vi "ActiView806-Lores.vi"() -> ()   [LabVIEW 2020] (continued)
                        i -> [w570]
                        n163 = call-poly <vilib>:"Read Key.vi"("section"=w578, "error in (no error)"=w588, "key"=w573, "refnum"=w589) -> ("error out"=w576:errorcluster, "value"=w584:string, "found?"=w583:bool, "refnum out"=w577:T19)  [unwired: 2 in, 2 out]
                        n164 = Decimal String To Number(string=w584) -> (number=w590:i32)  [unwired: 3 out]
                        n165 = Not(x=w583) -> (.not. x?=w586:bool)
                        n166 = Equal?(x="", y=w584) -> (x = y?=w585:bool)
                        n167 = To Byte Integer(number=w590) -> (8bit integer=w569:i8)
                        n168 = Equal To 0?(x=w570) -> (x = 0?=w580:bool)
                        n169 = Or(x=w586, y=w585) -> (x .or. y?=w582:bool)
                        n170 = Not Equal To 0?(x=w569) -> (x != 0?=w581:bool)
                        n171 = And(x=w581, y=w580) -> (x .and. y?=w579:bool)
                        n172 = case shown="True" w579 {
                          tunnel: w573 -> [_ w609]
                          tunnel: w578 -> [_ w608]
                          tunnel: w577 -> [w600 w607]
                          tunnel: w576 -> [w601 w606]
                          tunnel: w574 -> [_ w605]
                          tunnel: [w601 w604] -> w572
                          tunnel: [w600 w603] -> w575
                          frame False {
                          }
                          frame True {
                            n173 = call "Act_Warning.vi"() -> ("Warning?"=w602:bool)  [unwired: 1 out]
                            n174 = case shown="False" w602 {
                              tunnel: w609 -> [w615 _]
                              tunnel: w608 -> [w617 _]
                              tunnel: w607 -> [w616 w633]
                              tunnel: w606 -> [w610 w634]
                              tunnel: w605 -> [w614 _]
                              tunnel: [w612 w634] -> w604
                              tunnel: [w611 w633] -> w603
                              frame False {
                                n175 = flat-sequence {
                                tunnel: w617 -> [w628]
                                tunnel: w610 -> [w627]
                                tunnel: w616 -> [w626]
                                tunnel: w615 -> [w625]
                                tunnel: [w619] -> w613
                                tunnel: w614 -> [w632]
                                tunnel: w613 -> [w631]
                                tunnel: [w629] -> w612
                                tunnel: [w630] -> w611
                                frame #0 {
                                w618 = "0"  # No Warning
                                w620 = T18 1 items=["no dialog", "OK message", "continue or stop message", "OK message + warnings", "continue/stop + warnings"] ("type of dialog (OK msg:1)")
                                w623 = TRUE  # write configuration file? (T)
                                n176 = call-poly <vilib>:"Write Key.vi"("section"=w628, "error in (no error)"=w627, "value"=w618, "key"=w625, "refnum"=w626) -> ("error out"=w621:errorcluster, "refnum out"=w622:T19)  [unwired: 1 in, 4 out]
                                n177 = call <vilib>:"Close Config Data.vi"("error in (no error)"=w621, "write file if changed (T)"=w623, "refnum"=w622) -> ("error out"=w624:errorcluster)  [unwired: 8 out]
                                n178 = call <vilib>:"General Error Handler.vi"("type of dialog (OK msg:1)"=w620, "error in (no error)"=w624) -> ("error out"=w619:errorcluster)  [unwired: 1 in, 12 out]
                                }
                                frame #1 {
                                n179 = call <vilib>:"Open Config Data.vi"("error in (no error)"=w631, "configuration file path"=w632) -> ("error out"=w629:errorcluster, "refnum"=w630:T19)  [unwired: 7 in, 1 out]
                                }
                                }
                              }
                              frame True {
                              }
                            }
                          }
                        }
                        n180 = case shown="0, Default" w570 {
                          tunnel: w569 -> [w591 w595 w599]
                          tunnel: [w591 w592 w596] -> w571
                          frame 0, Default {
                          }
                          frame 4 {
                            # "LineWidth"
                            n181 = In Range and Coerce(upper limit=i8 1, x=w595, lower limit=i8 5) -> (coerced(x)=w592:i8)  [unwired: 1 out]
                          }
                          frame 5 {
                            # "Cursor"
                            n182 = In Range and Coerce(upper limit=i8 0, x=w599, lower limit=i8 1) -> (coerced(x)=w596:i8)  [unwired: 1 out]
                          }
                        }
                      }
                      n183 = Index Array(array=w557, index #1=2 ("index"), index #2=4 ("index")) -> (element #1=w554:i8, element #2=w558:i8)
                      n184 = To Unsigned Byte Integer(number=w558) -> (unsigned 8bit integer=w556:u8)
                      n185 = Or Array Elements(Boolean array=w561) -> (logical OR=w568:bool)
                    }
                    frame #1 {
                      # "Not Found"
                      # "Vbat is not a trace"
                      n186 = Decrement(x=w657) -> (x-1=w635:i32)
                      n187 = Add(x=w652, y=w642) -> (x+y=w641:i32)
                      n188 = Add(x=w652, y=w642) -> (x+y=w653:i32)
                      n189 = Add(x=w641, y=w657) -> (x+y=w640:i32)
                      n190 = Add(x=w640, y=w636) -> (x+y=w639:i32)
                      n191 = Add(x=w639, y=w650) -> (x+y=w655:i32)
                      n192 = for {
                        N: w653 -> [_]
                        tunnel: w649 -> [w751]
                        i -> [w750]
                        n193 = To Unsigned Long Integer(number=w750) -> (unsigned 32bit integer=w749:u32)
                        n194 = property on="Mon Chart" class="WFChart (strict)"("Active Plot"=w749, "Plot.Line Width"=w751) -> ()  [unwired: 2 in, 2 out]
                      }
                      n195 = for {
                        N: w652 -> [_]
                        tunnel: w649 -> [w748]
                        i -> [w747]
                        n196 = To Unsigned Long Integer(number=w747) -> (unsigned 32bit integer=w746:u32)
                        n197 = property on="Bip Chart" class="WFChart (strict)"("Active Plot"=w746, "Plot.Line Width"=w748) -> ()  [unwired: 2 in, 2 out]
                      }
                      n198 = To Unsigned Long Integer(number=w653) -> (unsigned 32bit integer=w671:u32)
                      n199 = To Unsigned Long Integer(number=w652) -> (unsigned 32bit integer=w660:u32)
                      n200 = To Unsigned Long Integer(number=w635) -> (unsigned 32bit integer=w659:u32)
                      n201 = To Unsigned Long Integer(number=w636) -> (unsigned 32bit integer=w651:u32)
                      n202 = To Unsigned Long Integer(number=w650) -> (unsigned 32bit integer=w656:u32)
                      n203 = Increment(x=w655) -> (x+1=w645:i32)
                      n204 = for {
                        N: w645 -> [w684]
                        shift-right: [w705] -> w644
                        shift-left: w647 -> [w707]
                        shift-right: [w704] -> w643
                        shift-left: w646 -> [w706]
                        tunnel: [w681] -> w637 mode=indexing
                        tunnel: [w693] -> w638 mode=indexing
                        tunnel: w642 -> [w685]
                        tunnel: w641 -> [w696]
                        tunnel: w648 -> [w680]
                        tunnel: w640 -> [w686]
                        tunnel: w639 -> [w673]
                        i -> [w675]
                        n205 = Increment(x=w675) -> (x+1=w683:i32)
                        n206 = Greater Or Equal?(x=w675, y=w696) -> (x >= y?=w701:bool)
                        n207 = Greater Or Equal?(x=w675, y=w685) -> (x >= y?=w703:bool)
                        n208 = Greater Or Equal?(x=w675, y=w686) -> (x >= y?=w687:bool)
                        n209 = Greater Or Equal?(x=w675, y=w673) -> (x >= y?=w674:bool)
                        n210 = Select(t=i8 1, s=w703, f=i8 0) -> (s? t:f=w702:i8)
                        n211 = Equal?(x=w684, y=w683) -> (x = y?=w676:bool)
                        n212 = Select(t=i8 2, s=w701, f=w702) -> (s? t:f=w690:i8)
                        n213 = Select(t=i8 3, s=w687, f=w690) -> (s? t:f=w689:i8)
                        n214 = Select(t=i8 4, s=w674, f=w689) -> (s? t:f=w678:i8)
                        n215 = Select(t=i8 5, s=w676, f=w678) -> (s? t:f=w679:i8)
                        n216 = case shown="5" w679 {
                          tunnel: [w711 w717 w723 w729 w735 "Trig" ("string")] -> w682
                          tunnel: w683 -> [w708 w715 w722 w726 w732 _]
                          tunnel: w685 -> [_ w714 _ _ _ _]
                          tunnel: w696 -> [_ _ w720 _ _ _]
                          tunnel: w686 -> [_ _ _ w724 _ _]
                          tunnel: w673 -> [_ _ _ _ w730 _]
                          frame 0, Default {
                            n217 = Number To Decimal String(number=w708) -> (decimal integer string=w709:string)  [unwired: 1 out]
                            n218 = Concatenate Strings("Chan" ("string"), w709) -> (w711:string)
                          }
                          frame 1 {
                            n219 = Subtract(x=w715, y=w714) -> (x-y=w712:i32)
                            n220 = Number To Decimal String(number=w712) -> (decimal integer string=w713:string)  [unwired: 1 out]
                            n221 = Concatenate Strings("Tou" ("string"), w713) -> (w717:string)
                          }
                          frame 2 {
                            n222 = Subtract(x=w722, y=w720) -> (x-y=w718:i32)
                            n223 = Number To Decimal String(number=w718) -> (decimal integer string=w719:string)  [unwired: 1 out]
                            n224 = Concatenate Strings("Aux" ("string"), w719) -> (w723:string)
                          }
                          frame 3 {
                            n225 = Subtract(x=w726, y=w724) -> (x-y=w725:i32)
                            n226 = Number To Decimal String(number=w725) -> (decimal integer string=w727:string)  [unwired: 1 out]
                            n227 = Concatenate Strings("Jazz" ("string"), w727) -> (w729:string)
                          }
                          frame 4 {
                            n228 = Subtract(x=w732, y=w730) -> (x-y=w731:i32)
                            n229 = Number To Decimal String(number=w731) -> (decimal integer string=w733:string)  [unwired: 1 out]
                            n230 = Concatenate Strings("Box" ("string"), w733) -> (w735:string)
                          }
                          frame 5 {
                          }
                        }
                        n231 = call-poly <vilib>:"Read Key.vi"("section"=w680, "error in (no error)"=w706, "key"=w682, "refnum"=w707) -> ("error out"=w704:errorcluster, "value"=w681:string, "found?"=w695:bool, "refnum out"=w705:T19)  [unwired: 2 in, 2 out]
                        n232 = Equal?(x="", y=w681) -> (x = y?=w691:bool)
                        n233 = Not(x=w695) -> (.not. x?=w694:bool)
                        n234 = Or(x=w691, y=w694) -> (x .or. y?=w693:bool)
                      }
                      n235 = property on="Mon Chart" class="WFChart (strict)"("Legend:Plots Shown"=w671) -> ()  [unwired: 2 in, 2 out]
                      n236 = property on="Bip Chart" class="WFChart (strict)"("Legend:Plots Shown"=w660) -> ()  [unwired: 2 in, 2 out]
                      n237 = property on="Aux Chart" class="WFChart (strict)"("Legend:Plots Shown"=w659) -> ()  [unwired: 2 in, 2 out]
                      n238 = property on="Jazz Chart" class="WFChart (strict)"("LegPlots"=w651) -> ()  [unwired: 2 in, 2 out]
                      n239 = property on="Ana Chart" class="WFChart (strict)"("Legend:Plots Shown"=w656) -> ()  [unwired: 2 in, 2 out]
                      n240 = Or Array Elements(Boolean array=w638) -> (logical OR=w654:bool)
                      n241 = Quotient & Remainder(x=w642, y=2) -> (floor(x/y)=w661:i32)  [unwired: 1 out]
                      n242 = case shown="False" w654 {
                        tunnel: w641 -> [w763 _]
                        tunnel: w652 -> [w762 _]
                        tunnel: w635 -> [w761 _]
                        tunnel: w642 -> [w760 _]
                        tunnel: w639 -> [w759 _]
                        tunnel: w650 -> [w758 _]
                        tunnel: w637 -> [w754 _]
                        tunnel: w636 -> [w756 _]
                        tunnel: w640 -> [w753 _]
                        frame False {
                          n243 = for {
                            N: w761 -> [_]
                            tunnel: w754 -> [w780]
                            tunnel: w763 -> [w781]
                            tunnel: [w779] -> w752 mode=indexing
                            i -> [w783]
                            n244 = Add(x=w781, y=w783) -> (x+y=w784:i32)
                            n245 = Index Array(array=w780, index=w784) -> (element=w785:string)
                            n246 = String Subset(string=w785, length (rest)=4 ("length (rest)")) -> (substring=w779:string)  [unwired: 1 out]
                          }
                          n247 = for {
                            N: w756 -> [_]
                            tunnel: w754 -> [w766]
                            tunnel: w753 -> [w767]
                            tunnel: [w765] -> w755 mode=indexing
                            i -> [w769]
                            n248 = Add(x=w767, y=w769) -> (x+y=w770:i32)
                            n249 = Index Array(array=w766, index=w770) -> (element=w771:string)
                            n250 = String Subset(string=w771, length (rest)=4 ("length (rest)")) -> (substring=w765:string)  [unwired: 1 out]
                          }
                          n251 = for {
                            N: w758 -> [_]
                            tunnel: w754 -> [w773]
                            tunnel: w759 -> [w774]
                            tunnel: [w772] -> w757 mode=indexing
                            i -> [w776]
                            n252 = Add(x=w774, y=w776) -> (x+y=w777:i32)
                            n253 = Index Array(array=w773, index=w777) -> (element=w778:string)
                            n254 = String Subset(string=w778, length (rest)=8 ("length (rest)")) -> (substring=w772:string)  [unwired: 1 out]
                          }
                          n255 = for {
                            N: w762 -> [w793]
                            tunnel: w754 -> [w798]
                            tunnel: w760 -> [w791]
                            tunnel: [w794] -> w764 mode=indexing
                            i -> [w789]
                            w786 = 4 ("length (rest)")
                            n256 = Increment(x=w789) -> (x+1=w788:i32)
                            n257 = Quotient & Remainder(x=w788, y=w793) -> (x-y*floor(x/y)=w787:i32)  [unwired: 1 out]
                            n258 = Add(x=w791, y=w789) -> (x+y=w792:i32)
                            n259 = Add(x=w791, y=w787) -> (x+y=w790:i32)
                            n260 = Index Array(array=w798, index=w792) -> (element=w800:string)
                            n261 = Index Array(array=w798, index=w790) -> (element=w799:string)
                            n262 = String Subset(string=w799, length (rest)=w786) -> (substring=w796:string)  [unwired: 1 out]
                            n263 = String Subset(string=w800, length (rest)=w786) -> (substring=w797:string)  [unwired: 1 out]
                            n264 = Concatenate Strings(w797, "-" ("string"), w796) -> (w794:string)
                          }
                          n265 = property on="AuxFree" class="LstBox (strict)"("Item Names"=w752) -> ()  [unwired: 2 in, 2 out]
                          n266 = property on="JazzFree" class="LstBox (strict)"("Item Names"=w755) -> ()  [unwired: 2 in, 2 out]
                          n267 = property on="AnaFree" class="LstBox (strict)"("Item Names"=w757) -> ()  [unwired: 2 in, 2 out]
                          n268 = property on="AnaOffset" class="Ring (strict)"("Strings []"=w757) -> ()  [unwired: 2 in, 2 out]
                          n269 = property on="BipFree" class="LstBox (strict)"("Item Names"=w764) -> ()  [unwired: 2 in, 2 out]
                        }
                        frame True {
                        }
                      }
                      n270 = Increment(x=w661) -> (x+1=w669:i32)
                      n271 = Increment(x=w661) -> (x+1=w664:i32)
                      n272 = for {
                        N: w636 -> [_]
                        tunnel: w649 -> [w739]
                        i -> [w738]
                        n273 = To Unsigned Long Integer(number=w738) -> (unsigned 32bit integer=w737:u32)
                        n274 = property on="Jazz Chart" class="WFChart (strict)"("Active Plot"=w737, "Plot.Line Width"=w739) -> ()  [unwired: 2 in, 2 out]
                      }
                      n275 = for {
                        N: w635 -> [_]
                        tunnel: w649 -> [w745]
                        i -> [w744]
                        n276 = To Unsigned Long Integer(number=w744) -> (unsigned 32bit integer=w743:u32)
                        n277 = property on="Aux Chart" class="WFChart (strict)"("Active Plot"=w743, "Plot.Line Width"=w745) -> ()  [unwired: 2 in, 2 out]
                      }
                      n278 = Increment(x=w664) -> (x+1=w670:i32)
                      n279 = Increment(x=w669) -> (x+1=w666:i32)
                      n280 = for {
                        N: w670 -> [w807]
                        tunnel: [w803] -> w663 mode=indexing
                        tunnel: [w801] -> w665
                        i -> [w810]
                        w801 = 1.0 ("X Scale.Offset and Multiplier:Offset")
                        w811 = 0.5 ("f")
                        n281 = Decrement(x=w807) -> (x-1=w806:i32)
                        n282 = Equal To 0?(x=w810) -> (x = 0?=w813:bool)
                        n283 = Equal?(x=w806, y=w810) -> (x = y?=w809:bool)
                        n284 = To Double Precision Float(number=w810) -> (double precision float=w812:dbl)
                        n285 = To Double Precision Float(number=w806) -> (double precision float=w805:dbl)
                        n286 = Select(t=w811, s=w813, f=w812) -> (s? t:f=w808:dbl)
                        n287 = Subtract(x=w805, y=w811) -> (x-y=w804:dbl)
                        n288 = Select(t=w804, s=w809, f=w808) -> (s? t:f=w802:dbl)
                        n289 = Subtract(x=w802, y=w801) -> (x-y=w803:dbl)
                      }
                      n290 = for {
                        N: w666 -> [w821]
                        tunnel: [w814] -> w667 mode=indexing
                        tunnel: [w816] -> w668
                        tunnel: w669 -> [w817]
                        i -> [w824]
                        w825 = 0.5 ("f")
                        n291 = Decrement(x=w821) -> (x-1=w820:i32)
                        n292 = Equal To 0?(x=w824) -> (x = 0?=w827:bool)
                        n293 = Equal?(x=w820, y=w824) -> (x = y?=w823:bool)
                        n294 = To Double Precision Float(number=w824) -> (double precision float=w826:dbl)
                        n295 = To Double Precision Float(number=w820) -> (double precision float=w819:dbl)
                        n296 = Select(t=w825, s=w827, f=w826) -> (s? t:f=w822:dbl)
                        n297 = Subtract(x=w819, y=w825) -> (x-y=w818:dbl)
                        n298 = To Double Precision Float(number=w817) -> (double precision float=w816:dbl)
                        n299 = Select(t=w818, s=w823, f=w822) -> (s? t:f=w815:dbl)
                        n300 = Decrement(x=w815) -> (x-1=w814:dbl)
                      }
                      n301 = for {
                        N: w650 -> [_]
                        tunnel: w649 -> [w742]
                        i -> [w741]
                        n302 = To Unsigned Long Integer(number=w741) -> (unsigned 32bit integer=w740:u32)
                        n303 = property on="Ana Chart" class="WFChart (strict)"("Active Plot"=w740, "Plot.Line Width"=w742) -> ()  [unwired: 2 in, 2 out]
                      }
                      n304 = property on="Offset Graph First Half" class="WFGraph (strict)"("X Scale.Marker Values[]"=w663) -> ()  [unwired: 2 in, 2 out]
                      n305 = property on="Offset Graph  Second Half" class="WFGraph (strict)"("X Scale.Marker Values[]"=w667) -> ()  [unwired: 2 in, 2 out]
                      n306 = Bundle By Name(cluster=w672, "All Labels"=w637) -> (w658:T8)
                      n307 = property on="Offset Graph First Half" class="WFGraph (strict)"("X Scale.Offset and Multiplier:Offset"=w665) -> ()  [unwired: 2 in, 2 out]
                      n308 = property on="Offset Graph  Second Half" class="WFGraph (strict)"("X Scale.Offset and Multiplier:Offset"=w668) -> ()  [unwired: 2 in, 2 out]
                    }
                    frame #2 {
                      # "not found"
                      n309 = for {
                        shift-right: [w961] -> w835
                        shift-left: w837 -> [w959]
                        shift-right: [w960] -> w834
                        shift-left: w836 -> [w958]
                        tunnel: [w957] -> w833 mode=indexing
                        tunnel: w830 -> [w956] mode=indexing
                        tunnel: [w950] -> w832 mode=indexing
                        tunnel: w829 -> [w949]
                        n310 = call-poly <vilib>:"Read Key.vi"("section"=w949, "error in (no error)"=w958, "key"=w956, "refnum"=w959) -> ("error out"=w960:errorcluster, "value"=w954:string, "found?"=w955:bool, "refnum out"=w961:T19)  [unwired: 2 in, 2 out]
                        n311 = Decimal String To Number(string=w954) -> (number=w957:i32)  [unwired: 3 out]
                        n312 = Not(x=w955) -> (.not. x?=w952:bool)
                        n313 = Equal?(x="", y=w954) -> (x = y?=w951:bool)
                        n314 = Or(x=w952, y=w951) -> (x .or. y?=w950:bool)
                      }
                      n315 = Or Array Elements(Boolean array=w832) -> (logical OR=w831:bool)
                      n316 = case shown="False" w831 {
                        tunnel: w833 -> [w946 _]
                        tunnel: w828 -> [w853 _]
                        frame False {
                          n317 = Index Array(array=w946) -> (element #1=w838:i32, element #2=w839:i32, element #3=w840:i32, element #4=w841:i32, element #5=w842:i32, element #6=w843:i32, element #7=w844:i32, element #8=w845:i32, element #9=w846:i32, element #10=w847:i32, element #11=w848:i32, element #12=w849:i32, element #13=w850:i32, element #14=w866:i32, element #15=w865:i32, element #16=w860:i32, element #17=w861:i32, element #18=w862:i32, element #19=w863:i32, element #20=w864:i32, element #21=w916:i32, element #22=w915:i32, element #23=w910:i32, element #24=w907:i32, element #25=w906:i32, element #26=w903:i32, element #27=w901:i32, element #28=w888:i32, element #29=w899:i32, element #30=w895:i32, element #31=w894:i32, element #32=w893:i32, element #33=w892:i32, element #34=w891:i32, element #35=w885:i32, element #36=w884:i32, element #37=w883:i32, element #38=w882:i32, element #39=w881:i32, element #40=w871:i32, element #41=w870:i32, element #42=w872:i32, element #43=w873:i32, element #44=w874:i32, element #45=w875:i32, element #46=w876:i32, element #47=w877:i32, element #48=w878:i32)  [unwired: 48 in]
                          n318 = case shown="0, Default" w853 {
                            tunnel: [i32[] [4] ("Disabled Items []") i32[] [] ("Disabled Items []")] -> w852
                            frame 0, Default {
                            }
                            frame 1 {
                            }
                          }
                          n319 = To Double Precision Float(number=w876) -> (double precision float=w926:dbl)
                          n320 = Not Equal To 0?(x=w881) -> (x != 0?=w930:bool)
                          n321 = Not Equal To 0?(x=w899) -> (x != 0?=w900:bool)
                          n322 = To Double Precision Float(number=w895) -> (double precision float=w898:dbl)
                          n323 = To Double Precision Float(number=w894) -> (double precision float=w897:dbl)
                          n324 = To Double Precision Float(number=w893) -> (double precision float=w896:dbl)
                          n325 = Not Equal To 0?(x=w871) -> (x != 0?=w869:bool)
                          n326 = To Byte Integer(number=w882) -> (8bit integer=w928:i8)
                          n327 = Not Equal To 0?(x=w901) -> (x != 0?=w902:bool)
                          n328 = To Double Precision Float(number=w874) -> (double precision float=w923:dbl)
                          n329 = To Byte Integer(number=w883) -> (8bit integer=w929:i8)
                          n330 = To Double Precision Float(number=w864) -> (double precision float=w936:dbl)
                          n331 = To Byte Integer(number=w891) -> (8bit integer=w914:i8)
                          n332 = Not Equal To 0?(x=w870) -> (x != 0?=w868:bool)
                          n333 = Not Equal To 0?(x=w873) -> (x != 0?=w924:bool)
                          n334 = To Byte Integer(number=w915) -> (8bit integer=w855:i8)
                          n335 = To Long Integer(number=w907) -> (32bit integer=w908:i32)
                          n336 = To Byte Integer(number=w910) -> (8bit integer=w909:i8)
                          n337 = To Byte Integer(number=w892) -> (8bit integer=w879:i8)
                          n338 = To Double Precision Float(number=w888) -> (double precision float=w890:dbl)
                          n339 = Not Equal To 0?(x=w875) -> (x != 0?=w922:bool)
                          n340 = To Byte Integer(number=w872) -> (8bit integer=w921:i8)
                          n341 = To Byte Integer(number=w884) -> (8bit integer=w913:i8)
                          n342 = To Byte Integer(number=w866) -> (8bit integer=w918:i8)
                          n343 = To Byte Integer(number=w860) -> (8bit integer=w937:i8)
                          n344 = Divide(x=w926, y=100.0) -> (x/y=w925:dbl)
                          n345 = To Double Precision Float(number=w903) -> (double precision float=w904:dbl)
                          n346 = Not Equal To 0?(x=w885) -> (x != 0?=w886:bool)
                          n347 = To Double Precision Float(number=w848) -> (double precision float=w941:dbl)
                          n348 = Not Equal To 0?(x=w877) -> (x != 0?=w912:bool)
                          n349 = Not Equal To 0?(x=w847) -> (x != 0?=w942:bool)
                          n350 = Not Equal To 0?(x=w906) -> (x != 0?=w905:bool)
                          n351 = To Byte Integer(number=w843) -> (8bit integer=w938:i8)
                          n352 = Not Equal To 0?(x=w863) -> (x != 0?=w932:bool)
                          n353 = To Quad Integer(1:w839) -> (0:w880:i64)
                          n354 = To Double Precision Float(number=w862) -> (double precision float=w933:dbl)
                          n355 = Not Equal To 0?(x=w840) -> (x != 0?=w911:bool)
                          n356 = To Double Precision Float(number=w846) -> (double precision float=w943:dbl)
                          n357 = To Byte Integer(number=w842) -> (8bit integer=w920:i8)
                          n358 = To Byte Integer(number=w844) -> (8bit integer=w945:i8)
                          n359 = Not Equal To 0?(x=w861) -> (x != 0?=w934:bool)
                          n360 = To Byte Integer(number=w865) -> (8bit integer=w867:i8)
                          n361 = Divide(x=w936, y=100.0) -> (x/y=w931:dbl)
                          n362 = Not Equal To 0?(x=w845) -> (x != 0?=w944:bool)
                          n363 = To Byte Integer(number=w916) -> (8bit integer=w917:i8)
                          n364 = Not Equal To 0?(x=w850) -> (x != 0?=w851:bool)
                          n365 = Divide(x=w890, y=100.0) -> (x/y=w887:dbl)
                          n366 = Divide(x=w941, y=100.0) -> (x/y=w939:dbl)
                          n367 = To Byte Integer(number=w849) -> (8bit integer=w919:i8)
                          n368 = To Byte Integer(number=w852) -> (8bit integer=w856:i8[])
                          n369 = property on="OffsetScale" class="Ring (strict)"("Disabled Items []"=w852) -> ()  [unwired: 2 in, 2 out]
                          n370 = local write "RecTimeLimit"(w841) -> ()
                          n371 = local write "MonHPfreq"(w939) -> ()
                          n372 = local write "FileLimit"(w880) -> ()
                          n373 = local write "FileAppend"(w911) -> ()
                          n374 = local write "Decimation"(w920) -> ()
                          n375 = local write "MonScale"(w945) -> ()
                          n376 = local write "MonLP"(w944) -> ()
                          n377 = local write "MonLPfreq"(w943) -> ()
                          n378 = local write "MonHP"(w942) -> ()
                          n379 = local write "BipHPfreq"(w931) -> ()
                          n380 = local write "AvgLPfreq"(w904) -> ()
                          n381 = local write "ScreenLength"(w838) -> ()
                          n382 = local write "TrigCode"(w867) -> ()
                          n383 = local write "BipScale"(w937) -> ()
                          n384 = local write "BipLP"(w934) -> ()
                          n385 = local write "BipLPfreq"(w933) -> ()
                          n386 = local write "BipHP"(w932) -> ()
                          n387 = local write "AvgTrigLog"(w909) -> ()
                          n388 = local write "AvgHPfreq"(w887) -> ()
                          n389 = local write "AvgAutoscale"(w900) -> ()
                          n390 = local write "TempScale"(w928) -> ()
                          n391 = local write "AnaHPfreq"(w925) -> ()
                          n392 = local write "Channels"(w919) -> ()
                          n393 = local write "AddTP"(w851) -> ()
                          n394 = local write "AvgSweep"(w908) -> ()
                          n395 = local write "AvgLP"(w905) -> ()
                          n396 = local write "AvgHP"(w902) -> ()
                          n397 = local write "AvgScale"(w898) -> ()
                          n398 = local write "AvgAbsReject"(w897) -> ()
                          n399 = local write "AvgRelReject"(w896) -> ()
                          n400 = local write "GsrScale"(w879) -> ()
                          n401 = local write "ErgoScale"(w914) -> ()
                          n402 = local write "ErgoLP"(w886) -> ()
                          n403 = local write "RespScale"(w913) -> ()
                          n404 = local write "PletScale"(w929) -> ()
                          n405 = local write "AnaScale"(w921) -> ()
                          n406 = local write "AnaLP"(w924) -> ()
                          n407 = local write "AnaLPfreq"(w923) -> ()
                          n408 = local write "AnaHP"(w922) -> ()
                          n409 = local write "Buffer"(w938) -> ()
                          n410 = local write "Reference"(w918) -> ()
                          n411 = local write "Offset"(w917) -> ()
                          n412 = local write "AuxReset"(w930) -> ()
                          n413 = local write "JazzOn"(w869) -> ()
                          n414 = local write "AnaReset"(w912) -> ()
                          n415 = local write "AnaOffset"(w878) -> ()
                          n416 = local write "JazzReset"(w868) -> ()
                          n417 = Search 1D Array(1D array=w856, element=w855) -> (index of element=w857:i32)  [unwired: 1 out]
                          n418 = Less Than 0?(x=w857) -> (x < 0?=w858:bool)
                          n419 = Select(t=w855, s=w858, f=i8 3) -> (s? t:f=w854:i8)
                          n420 = local write "OffsetScale"(w854) -> ()
                        }
                        frame True {
                        }
                      }
                    }
                    frame #3 {
                      w962 = FALSE  # Not found
                      # "not found"
                      n421 = for {
                        tunnel: w969 -> [w977] mode=indexing
                        shift-right: [w981] -> w964
                        shift-left: w967 -> [w984]
                        shift-right: [w982] -> w965
                        shift-left: w968 -> [w985]
                        tunnel: w966 -> [w983]
                        shift-right: [w970] -> w963
                        shift-left: w962 -> [w972]
                        i -> [w976]
                        n422 = call-poly <vilib>:"Read Key.vi"("section"=w983, "error in (no error)"=w984, "key"=w977, "refnum"=w985) -> ("error out"=w981:errorcluster, "value"=w978:string, "found?"=w979:bool, "refnum out"=w982:T19)  [unwired: 2 in, 2 out]
                        n423 = Not(x=w979) -> (.not. x?=w973:bool)
                        n424 = Equal?(x="", y=w978) -> (x = y?=w974:bool)
                        n425 = call "CFGtoArray.vi"("Cofiguration String"=w978) -> ("Selector Array"=w975:i32[])
                        n426 = Or(x=w973, y=w974) -> (x .or. y?=w971:bool)
                        n427 = case shown="False" w971 {
                          tunnel: w976 -> [w987 _]
                          tunnel: w975 -> [w986 _]
                          frame False {
                            n428 = case shown="0, Default" w987 {
                              tunnel: w986 -> [w988 w989 w990 w991 w993 w994 w996 w997 w998 w999 w1000]
                              frame 0, Default {
                                n429 = local write "MonFree"(w988) -> ()
                              }
                              frame 1 {
                                n430 = local write "RefFree"(w989) -> ()
                              }
                              frame 2 {
                                n431 = local write "BipFree"(w990) -> ()
                              }
                              frame 3 {
                                n432 = local write "AvgTrigSel"(w991) -> ()
                              }
                              frame 4 {
                                n433 = Index Array(array=w993) -> (element=w992:i32)  [unwired: 1 in]
                                n434 = local write "MonFreeAvg1"(w992) -> ()
                              }
                              frame 5 {
                                n435 = local write "RefFreeAvg1"(w994) -> ()
                              }
                              frame 6 {
                                n436 = Index Array(array=w996) -> (element=w995:i32)  [unwired: 1 in]
                                n437 = local write "MonFreeAvg2"(w995) -> ()
                              }
                              frame 7 {
                                n438 = local write "RefFreeAvg2"(w997) -> ()
                              }
                              frame 8 {
                                n439 = local write "AuxFree"(w998) -> ()
                              }
                              frame 9 {
                                n440 = local write "JazzFree"(w999) -> ()
                              }
                              frame 10 {
                                n441 = local write "AnaFree"(w1000) -> ()
                              }
                            }
                          }
                          frame True {
                          }
                        }
                        n442 = Or(x=w972, y=w971) -> (x .or. y?=w970:bool)
                      }
                    }
                    frame #4 {
                      w1008 = TRUE  # read raw string? (F)
                      # "Not Found"
                      n443 = Array Size(array=w1004) -> (size(s)=w1007:i32)
                      n444 = Decrement(x=w1007) -> (x-1=w1005:i32)
                      n445 = Decrement(x=w1007) -> (x-1=w1006:i32)
                      n446 = Index Array(array=w1004, index=w1006) -> (element=w1003:string)
                      n447 = for {
                        N: w1005 -> [_]
                        shift-right: [w1036] -> w1012
                        shift-left: w1024 -> [w1035]
                        shift-right: [w1037] -> w1011
                        shift-left: w1023 -> [w1034]
                        tunnel: [w1025] -> w1022 mode=indexing
                        tunnel: [w1028] -> w1021 mode=indexing
                        tunnel: w1018 -> [w1027]
                        tunnel: w1004 -> [w1026] mode=indexing
                        n448 = call-poly <vilib>:"Read Key.vi"("section"=w1027, "error in (no error)"=w1034, "key"=w1026, "refnum"=w1035) -> ("error out"=w1037:errorcluster, "value"=w1030:string, "found?"=w1029:bool, "refnum out"=w1036:T19)  [unwired: 2 in, 2 out]
                        n449 = Not(x=w1029) -> (.not. x?=w1032:bool)
                        n450 = Equal?(x="", y=w1030) -> (x = y?=w1031:bool)
                        n451 = Decimal String To Number(string=w1030) -> (number=w1025:i32)  [unwired: 3 out]
                        n452 = Or(x=w1032, y=w1031) -> (x .or. y?=w1028:bool)
                      }
                      n453 = call-poly <vilib>:"Read Key.vi"("read raw string? (F)"=w1008, "section"=w1018, "error in (no error)"=w1011, "key"=w1003, "refnum"=w1012) -> ("error out"=w1001:errorcluster, "value"=w1009:string, "found?"=w1017:bool, "refnum out"=w1002:T19)  [unwired: 1 in, 2 out]
                      n454 = Not(x=w1017) -> (.not. x?=w1016:bool)
                      n455 = Equal?(x="", y=w1009) -> (x = y?=w1019:bool)
                      n456 = String To Path(string=w1009) -> (path=w1010:path)
                      n457 = Or(x=w1016, y=w1019) -> (x .or. y?=w1013:bool)
                      n458 = Or Array Elements(Boolean array=w1021) -> (logical OR=w1014:bool)
                      n459 = Or(x=w1014, y=w1013) -> (x .or. y?=w1015:bool)
                    }
                    frame #5 {
                      # "Not Found"
                      n460 = for {
                        shift-right: [w1073] -> w1042
                        shift-left: w1046 -> [w1072]
                        shift-right: [w1074] -> w1041
                        shift-left: w1045 -> [w1071]
                        tunnel: [w1062] -> w1039 mode=indexing
                        tunnel: [w1065] -> w1040 mode=indexing
                        tunnel: w1043 -> [w1064]
                        tunnel: w1044 -> [w1063] mode=indexing
                        n461 = call-poly <vilib>:"Read Key.vi"("section"=w1064, "error in (no error)"=w1071, "key"=w1063, "refnum"=w1072) -> ("error out"=w1074:errorcluster, "value"=w1067:string, "found?"=w1066:bool, "refnum out"=w1073:T19)  [unwired: 2 in, 2 out]
                        n462 = Not(x=w1066) -> (.not. x?=w1069:bool)
                        n463 = Equal?(x="", y=w1067) -> (x = y?=w1068:bool)
                        n464 = Decimal String To Number(string=w1067) -> (number=w1062:i32)  [unwired: 3 out]
                        n465 = Or(x=w1069, y=w1068) -> (x .or. y?=w1065:bool)
                      }
                      n466 = Or Array Elements(Boolean array=w1040) -> (logical OR=w1038:bool)
                      n467 = case shown="False" w1038 {
                        tunnel: w1039 -> [w1061 _]
                        frame False {
                          n468 = Index Array(array=w1061) -> (element #1=w1060:i32, element #2=w1059:i32, element #3=w1058:i32, element #4=w1057:i32, element #5=w1048:i32, element #6=w1049:i32, element #7=w1050:i32)  [unwired: 7 in]
                          n469 = Not Equal To 0?(x=w1058) -> (x != 0?=w1054:bool)
                          n470 = Not Equal To 0?(x=w1048) -> (x != 0?=w1047:bool)
                          n471 = Not Equal To 0?(x=w1050) -> (x != 0?=w1051:bool)
                          n472 = To Byte Integer(number=w1059) -> (8bit integer=w1053:i8)
                          n473 = Not Equal To 0?(x=w1057) -> (x != 0?=w1055:bool)
                          n474 = Not Equal To 0?(x=w1049) -> (x != 0?=w1056:bool)
                          n475 = To Unsigned Word Integer(number=w1060) -> (unsigned 16bit integer=w1052:u16)
                          n476 = local write "LocalPort"(w1052) -> ()
                          n477 = local write "TCPaddTP"(w1054) -> ()
                          n478 = local write "TCPaddAnas"(w1056) -> ()
                          n479 = local write "TCPaddTrig"(w1051) -> ()
                          n480 = local write "TCPsubset"(w1053) -> ()
                          n481 = local write "TCPaddSens"(w1055) -> ()
                          n482 = local write "TCPaddJazz"(w1047) -> ()
                        }
                        frame True {
                        }
                      }
                    }
                  }
                  n483 = Compound Arithmetic op=OR(w516, w517, w515, w530, w540, w519) -> (w529:bool)
                  n484 = Build Array(w529) -> (w542:bool[])
                  n485 = Boolean Array To Number(Boolean array=w542) -> (number=w541:u32)
                  n486 = call "Act_ConfigError.vi"("Error Code In"=w541, "error in (no error)"=w545) -> ("[user-defined descriptions]"=w543:string[], "[user-defined codes]"=w544:i32[], "error out"=w546:errorcluster)
                  n487 = call <vilib>:"Close Config Data.vi"("error in (no error)"=w546, "write file if changed (T)"=FALSE ("write configuration file? (T)"), "refnum"=w550) -> ("error out"=w552:errorcluster)  [unwired: 8 out]
                  n488 = call <vilib>:"General Error Handler.vi"("[user-defined codes]"=w544, "[user-defined descriptions]"=w543, "type of dialog (OK msg:1)"=w523, "error in (no error)"=w552) -> ()  [unwired: 1 in, 11 out]
                }
                frame True {
                }
              }
            }
            frame 2 {
              n489 = Current VI's Path() -> (path=w1112:path)
              n490 = Strip Path(path=w1112) -> (stripped path=w1111:path)  [unwired: 1 out]
              n491 = case shown="True" w1088 {
                tunnel: w1111 -> [w1425 w1427]
                tunnel: [w1425 w1426] -> w1110
                frame False {
                }
                frame True {
                  n492 = Strip Path(path=w1427) -> (stripped path=w1426:path)  [unwired: 1 out]
                }
              }
              n493 = File Dialog(4:w1085, 6:w1086, 7:"Enter filename:" ("prompt"), 9:w1086, 11:w1110) -> (0:w1087:errorcluster, 1:w1107:bool, 3:w1108:path)  [unwired: 1 in, 2 out]
              n494 = case shown="False" w1107 {
                tunnel: w1108 -> [w1117 _]
                tunnel: w1106 -> [w1276 _]
                tunnel: w1105 -> [w1165 _]
                tunnel: w1104 -> [w1166 _]
                tunnel: w1103 -> [w1157 _]
                tunnel: w1102 -> [w1283 _]
                tunnel: w1101 -> [w1282 _]
                tunnel: w1100 -> [w1281 _]
                tunnel: w1099 -> [w1237 _]
                tunnel: w1098 -> [w1234 _]
                tunnel: w1097 -> [w1280 _]
                tunnel: w1096 -> [w1187 _]
                tunnel: w1095 -> [w1253 _]
                tunnel: w1094 -> [w1256 _]
                tunnel: w1093 -> [w1255 _]
                tunnel: w1092 -> [w1248 _]
                tunnel: w1091 -> [w1190 _]
                tunnel: w1090 -> [w1240 _]
                tunnel: w1089 -> [w1191 _]
                tunnel: w1087 -> [w1116 _]
                tunnel: w1084 -> [w1162 _]
                tunnel: w1083 -> [w1163 _]
                frame False {
                  w1246 = TRUE  # write raw string? (F)
                  w1251 = i8 1  # New CFG has warning
                  w1254 = T18 1 items=["no dialog", "OK message", "continue or stop message", "OK message + warnings", "continue/stop + warnings"] ("type of dialog (OK msg:1)")
                  w1284 = TRUE  # write configuration file?
                  n495 = call <vilib>:"Open Config Data.vi"("error in (no error)"=w1116, "configuration file path"=w1117) -> ("error out"=w1114:errorcluster, "refnum"=w1115:T19)  [unwired: 7 in, 1 out]
                  n496 = Replace Array Subset(array=w1253, new element=w1251) -> (w1252:i8[])  [unwired: 1 in]
                  n497 = Add(x=w1157, y=w1283) -> (x+y=w1158:i32)
                  n498 = Unbundle By Name(w1281) -> ("All Labels"=w1169:string[])
                  n499 = Add(x=w1158, y=w1282) -> (x+y=w1159:i32)
                  n500 = for {
                    shift-right: [w1403] -> w1168
                    shift-left: w1115 -> [w1406]
                    shift-right: [w1404] -> w1170
                    shift-left: w1114 -> [w1405]
                    tunnel: w1256 -> [w1402]
                    tunnel: w1252 -> [w1401] mode=indexing
                    tunnel: w1255 -> [w1399] mode=indexing
                    n501 = Number To Decimal String(number=w1401) -> (decimal integer string=w1400:string)  [unwired: 1 out]
                    n502 = call-poly <vilib>:"Write Key.vi"("section"=w1402, "error in (no error)"=w1405, "value"=w1400, "key"=w1399, "refnum"=w1406) -> ("error out"=w1404:errorcluster, "refnum out"=w1403:T19)  [unwired: 1 in, 4 out]
                  }
                  n503 = Add(x=w1159, y=w1163) -> (x+y=w1160:i32)
                  n504 = Add(x=w1160, y=w1162) -> (x+y=w1161:i32)
                  n505 = Increment(x=w1161) -> (x+1=w1167:i32)
                  n506 = for {
                    N: w1167 -> [w1325]
                    shift-right: [w1312] -> w1164
                    shift-left: w1168 -> [w1314]
                    shift-right: [w1311] -> w1171
                    shift-left: w1170 -> [w1315]
                    tunnel: w1157 -> [w1326]
                    tunnel: w1158 -> [w1332]
                    tunnel: w1166 -> [w1313]
                    tunnel: w1159 -> [w1327]
                    tunnel: w1160 -> [w1317]
                    tunnel: w1169 -> [w1310] mode=indexing
                    i -> [w1319]
                    n507 = Increment(x=w1319) -> (x+1=w1324:i32)
                    n508 = Greater Or Equal?(x=w1319, y=w1332) -> (x >= y?=w1337:bool)
                    n509 = Greater Or Equal?(x=w1319, y=w1326) -> (x >= y?=w1339:bool)
                    n510 = Greater Or Equal?(x=w1319, y=w1327) -> (x >= y?=w1328:bool)
                    n511 = Greater Or Equal?(x=w1319, y=w1317) -> (x >= y?=w1318:bool)
                    n512 = Select(t=i8 1, s=w1339, f=i8 0) -> (s? t:f=w1338:i8)
                    n513 = Equal?(x=w1325, y=w1324) -> (x = y?=w1320:bool)
                    n514 = Select(t=i8 2, s=w1337, f=w1338) -> (s? t:f=w1331:i8)
                    n515 = Select(t=i8 3, s=w1328, f=w1331) -> (s? t:f=w1330:i8)
                    n516 = Select(t=i8 4, s=w1318, f=w1330) -> (s? t:f=w1322:i8)
                    n517 = Select(t=i8 5, s=w1320, f=w1322) -> (s? t:f=w1323:i8)
                    n518 = case shown="5" w1323 {
                      tunnel: [w1343 w1349 w1355 w1361 w1367 "Trig" ("string")] -> w1316
                      tunnel: w1324 -> [w1340 w1347 w1354 w1358 w1364 _]
                      tunnel: w1326 -> [_ w1346 _ _ _ _]
                      tunnel: w1332 -> [_ _ w1352 _ _ _]
                      tunnel: w1327 -> [_ _ _ w1356 _ _]
                      tunnel: w1317 -> [_ _ _ _ w1362 _]
                      frame 0, Default {
                        n519 = Number To Decimal String(number=w1340) -> (decimal integer string=w1341:string)  [unwired: 1 out]
                        n520 = Concatenate Strings("Chan" ("string"), w1341) -> (w1343:string)
                      }
                      frame 1 {
                        n521 = Subtract(x=w1347, y=w1346) -> (x-y=w1344:i32)
                        n522 = Number To Decimal String(number=w1344) -> (decimal integer string=w1345:string)  [unwired: 1 out]
                        n523 = Concatenate Strings("Tou" ("string"), w1345) -> (w1349:string)
                      }
                      frame 2 {
                        n524 = Subtract(x=w1354, y=w1352) -> (x-y=w1350:i32)
                        n525 = Number To Decimal String(number=w1350) -> (decimal integer string=w1351:string)  [unwired: 1 out]
                        n526 = Concatenate Strings("Aux" ("string"), w1351) -> (w1355:string)
                      }
                      frame 3 {
                        n527 = Subtract(x=w1358, y=w1356) -> (x-y=w1357:i32)
                        n528 = Number To Decimal String(number=w1357) -> (decimal integer string=w1359:string)  [unwired: 1 out]
                        n529 = Concatenate Strings("Jazz" ("string"), w1359) -> (w1361:string)
                      }
                      frame 4 {
                        n530 = Subtract(x=w1364, y=w1362) -> (x-y=w1363:i32)
                        n531 = Number To Decimal String(number=w1363) -> (decimal integer string=w1365:string)  [unwired: 1 out]
                        n532 = Concatenate Strings("Box" ("string"), w1365) -> (w1367:string)
                      }
                      frame 5 {
                      }
                    }
                    n533 = call-poly <vilib>:"Write Key.vi"("section"=w1313, "error in (no error)"=w1315, "value"=w1310, "key"=w1316, "refnum"=w1314) -> ("error out"=w1311:errorcluster, "refnum out"=w1312:T19)  [unwired: 2 in, 3 out]
                  }
                  n534 = local read "AvgAbsReject"() -> (w1226:dbl)
                  n535 = local read "ScreenLength"() -> (w1118:i32)
                  n536 = local read "AvgAutoscale"() -> (w1228:bool)
                  n537 = local read "RecTimeLimit"() -> (w1121:i32)
                  n538 = local read "AvgRelReject"() -> (w1227:dbl)
                  n539 = local read "MonHPfreq"() -> (w1302:dbl)
                  n540 = local read "FileAppend"() -> (w1242:bool)
                  n541 = local read "OffsetScale"() -> (w1275:i8)
                  n542 = local read "AvgTrigLog"() -> (w1232:i8)
                  n543 = local read "Decimation"() -> (w1286:i8)
                  n544 = local read "MonLPfreq"() -> (w1305:dbl)
                  n545 = local read "AvgHPfreq"() -> (w1208:dbl)
                  n546 = local read "AnaHPfreq"() -> (w1262:dbl)
                  n547 = local read "AvgLPfreq"() -> (w1220:dbl)
                  n548 = local read "TempScale"() -> (w1273:i8)
                  n549 = local read "AvgSweep"() -> (w1231:i32)
                  n550 = local read "AnaLPfreq"() -> (w1269:dbl)
                  n551 = local read "Reference"() -> (w1298:i8)
                  n552 = local read "BipHPfreq"() -> (w1292:dbl)
                  n553 = local read "RespScale"() -> (w1257:i8)
                  n554 = local read "AnaOffset"() -> (w1154:i32)
                  n555 = local read "MonScale"() -> (w1308:i8)
                  n556 = local read "ErgoScale"() -> (w1258:i8)
                  n557 = local read "JazzReset"() -> (w1143:bool)
                  n558 = local read "BipLPfreq"() -> (w1291:dbl)
                  n559 = local read "AuxReset"() -> (w1272:bool)
                  n560 = local read "AnaReset"() -> (w1244:bool)
                  n561 = local read "Channels"() -> (w1299:i8)
                  n562 = local read "TrigCode"() -> (w1261:i8)
                  n563 = local read "AvgScale"() -> (w1225:dbl)
                  n564 = local read "AnaScale"() -> (w1270:i8)
                  n565 = local read "PletScale"() -> (w1274:i8)
                  n566 = local read "GsrScale"() -> (w1172:i8)
                  n567 = local read "BipScale"() -> (w1296:i8)
                  n568 = local read "FileLimit"() -> (w1241:i64)
                  n569 = local read "MonHP"() -> (w1303:bool)
                  n570 = local read "JazzOn"() -> (w1145:bool)
                  n571 = local read "MonLP"() -> (w1307:bool)
                  n572 = local read "ErgoLP"() -> (w1180:bool)
                  n573 = local read "AvgHP"() -> (w1229:bool)
                  n574 = local read "AnaHP"() -> (w1266:bool)
                  n575 = local read "AddTP"() -> (w1131:bool)
                  n576 = local read "Offset"() -> (w1287:i8)
                  n577 = local read "AvgLP"() -> (w1230:bool)
                  n578 = local read "AnaLP"() -> (w1267:bool)
                  n579 = local read "Buffer"() -> (w1285:i8)
                  n580 = local read "BipHP"() -> (w1289:bool)
                  n581 = local read "BipLP"() -> (w1294:bool)
                  n582 = Boolean To (0,1)(Boolean=w1294) -> (0, 1=w1295:i16)
                  n583 = Boolean To (0,1)(Boolean=w1289) -> (0, 1=w1290:i16)
                  n584 = Boolean To (0,1)(Boolean=w1307) -> (0, 1=w1306:i16)
                  n585 = To Long Integer(number=w1298) -> (32bit integer=w1297:i32)
                  n586 = Boolean To (0,1)(Boolean=w1131) -> (0, 1=w1132:i16)
                  n587 = Boolean To (0,1)(Boolean=w1303) -> (0, 1=w1304:i16)
                  n588 = Boolean To (0,1)(Boolean=w1242) -> (0, 1=w1243:i16)
                  n589 = To Long Integer(number=w1291) -> (32bit integer=w1135:i32)
                  n590 = Boolean To (0,1)(Boolean=w1272) -> (0, 1=w1271:i16)
                  n591 = To Long Integer(number=w1241) -> (32bit integer=w1119:i32)
                  n592 = To Long Integer(number=w1296) -> (32bit integer=w1137:i32)
                  n593 = Boolean To (0,1)(Boolean=w1180) -> (0, 1=w1181:i16)
                  n594 = Boolean To (0,1)(Boolean=w1145) -> (0, 1=w1146:i16)
                  n595 = To Long Integer(number=w1308) -> (32bit integer=w1124:i32)
                  n596 = Multiply(x=w1302, y=100.0) -> (x*y=w1300:dbl)
                  n597 = To Long Integer(number=w1295) -> (32bit integer=w1136:i32)
                  n598 = Boolean To (0,1)(Boolean=w1143) -> (0, 1=w1147:i16)
